vi "Clear Audio Device.vi"(8 "error in (no error)":errorcluster, 11 "Audio Device Refnum In":T1) -> (0 "error out":errorcluster)   [LabVIEW 2020, in "G-Audio.lvlib"]
doc: "Clear the audio device and free any associated resources."
uses:
  G-Audio.lvlib
  Controls/Audio Device Refnum.ctl
  <vilib>/Utility/error.llb/Error Cluster From Error Code.vi
  lib/g_audio_x86.dll
  lib/g_audio_x64.dll
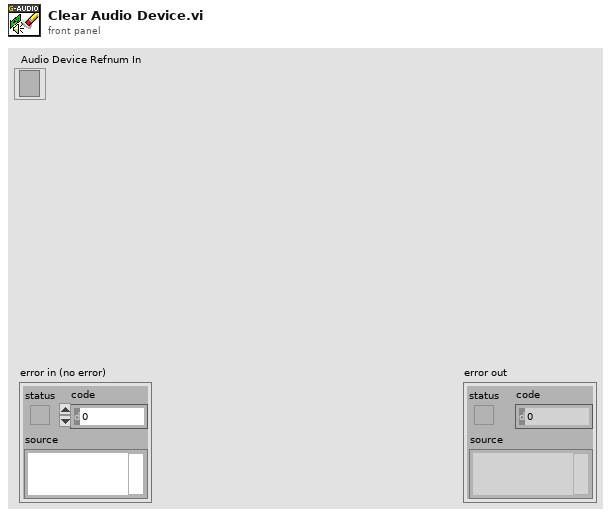
[diagram p1: front panel]
types:
  T1 = typedef "G-Audio.lvlib/Audio Device Refnum.ctl" = refnum<file>
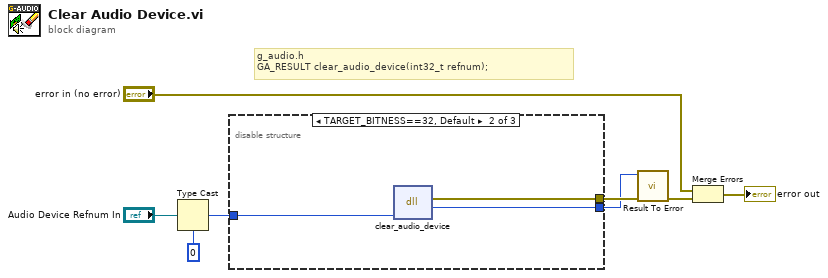
[diagram p0: block diagram]
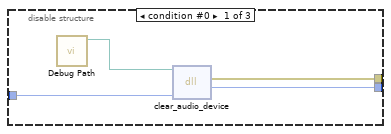
[diagram p2: hidden frame]
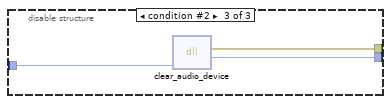
[diagram p3: hidden frame]
diagram:
  # "g_audio.h\nGA_RESULT clear_audio_device(int32_t refnum);"
  n1 = Type Cast(type=0, x="Audio Device Refnum In") -> (*(type *) &x=w4:i32)
  n2 = disable-structure shown="TARGET_BITNESS==32, Default" {
    disable-tunnel: [w11 w15 w18] -> w7
    disable-tunnel: [w10 w14 w17] -> w6
    disable-tunnel: w4 -> [w9 w13 w16]
    frame condition #0 {
      n3 = call "Debug Path.vi"() -> ("Debug Path"=w12:path)  [unwired: 11 in]
      n4 = dll-call lib="?" fn="clear_audio_device"(path in=w12, "refnum"=w9) -> (error out=w11:errorcluster, "result"=w10:i32)  [unwired: 3 in, 1 out]
    }
    frame condition #1 (active) {
      n5 = dll-call lib="C:/github/dataflowg/g-audio/src/LabVIEW/G-Audio/lib/g_audio_x86.*" fn="clear_audio_device"("refnum"=w13) -> (error out=w15:errorcluster, "result"=w14:i32)  [unwired: 4 in, 1 out]
    }
    frame condition #2 {
      n6 = dll-call lib="C:/github/dataflowg/g-audio/src/LabVIEW/G-Audio/lib/g_audio_x64.*" fn="clear_audio_device"("refnum"=w16) -> (error out=w18:errorcluster, "result"=w17:i32)  [unwired: 4 in, 1 out]
    }
  }
  n7 = call "Result To Error.vi"("error in (no error)"=w7, "Result Code"=w6) -> ("error out"=w8:errorcluster)  [unwired: 9 in]
  n8 = Merge Errors("error in (no error)", w8) -> (→"error out":errorcluster)
